vi "runTestScenario.vi"(8 "error in (no error)":errorcluster, 11 "Digital Output Test  in":refnum<class "Digital Output Test.lvclass">) -> (0 "error out":errorcluster, 2 "TestExecution":T1, 3 "Digital Output Test out":refnum<class "Digital Output Test.lvclass">)   [LabVIEW 2015, in "Digital Output Test.lvclass"]
uses:
  Digital Output Test.lvclass
  Typedefs/TestExecution.ctl
  Typedefs/WriteLogMessageInput.ctl
  Typedefs/TestScenarioTypes.ctl
  Typedefs/PassFailTest.ctl
  Digital Output Test.lvclass/Digital Output Test.ctl
  Model/TestLog/ITestLog/ITestLog.lvclass
  Model/ConfigureILCStrategy/IConfigureILCStrategy/IConfigureILCStrategy.lvclass
  Typedefs/ILCBTTypedefs.lvlib
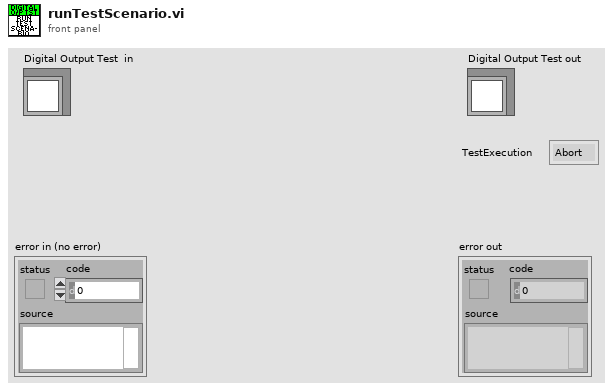
[diagram p1: front panel]
types:
  T1 = typedef "ILCBTTypedefs.lvlib/TestExecution.ctl" = enum16{"Abort", "Continue"}
  T2 = typedef "ILCBTTypedefs.lvlib/WriteLogMessageInput.ctl" = cluster{"Test Scenario":T3, "Description":string, "Actual Value":string, "Data File":string, "Result":T4}
  T3 = typedef "ILCBTTypedefs.lvlib/TestScenarioTypes.ctl" = enum16{"+3.3VA Supply Test", "+3.3VD Supply Test", "+5VA Supply Test", "+5VD Supply Test", "Unique ID Test", "TEDS Status Test", "LIMSW1_TTL Low Test", "LIMSW1_TTL High Test", "LIMSW2_TTL Low Test", "LIMSW2_TTL High Test", "Tachometer Test", "SSR_TTL Low Test", "SSR_TTL High Test", "SM_CW Low Test", "SM_CW High Test", "SM_CCW Low Test", "SM_CCW High Test", "SM_GPI Low Test", "SM_GPI High Test", "CW Motion Without Limit Test", "CW Motion With Limit Test", "CW Motion With Limit Interruption Test", "CW Motion on CCW Limit Test", "CCW Motion Without Limit Test", "CCW Motion With Limit Test", "CCW Motion With Limit Interruption Test", "CCW Motion on CW Limit Test", "RS232-TXD Low Test", "RS232-TXD High Test", "RS232-RTS Low Test", "RS232-RTS High Test", "RS232-RXD Low Test", "RS232-RXD High Test", "RS232-CTS Low Test", "RS232-CTS High Test", "Out_SS Low Test", "Out_SS High Test", "Out_SDI Low Test", "Out_SDI High Test", "Out_SCLK Low Test", "Out_SCLK High Test", "Reset Low Test", "Reset High Test", "1 Channel ADC Test", "3 Channel ADC Test", "5 Channel ADC Test", "Vref Test", "ROT Test", "DAC1 Test", "DAC2 Test", "DAC3 Test", "DAC4 Test", "BIAS Test", "EXC1 Test", "EXC2 Test", "EXC3 Test", "EXC4 Test"}
  T4 = typedef "ILCBTTypedefs.lvlib/PassFailTest.ctl" = enum16{"Fail", "Pass", "NA"}
  T5 = typedef "ILCBTTypedefs.lvlib/Digital Signal Level.ctl" = enum16{"Low", "High"}
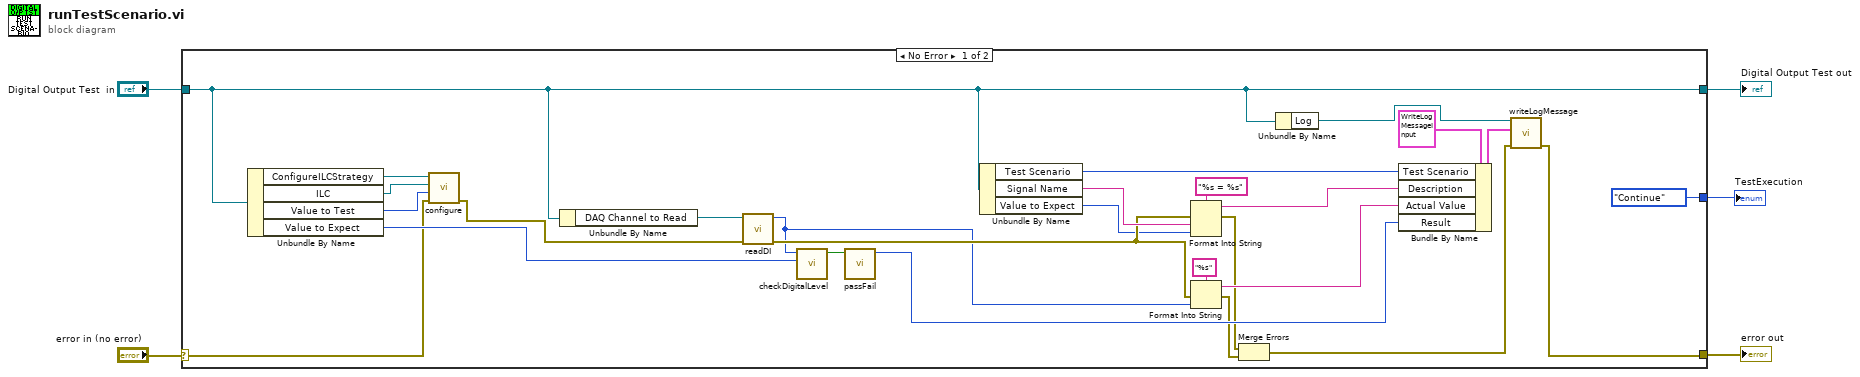
[diagram p0: block diagram]
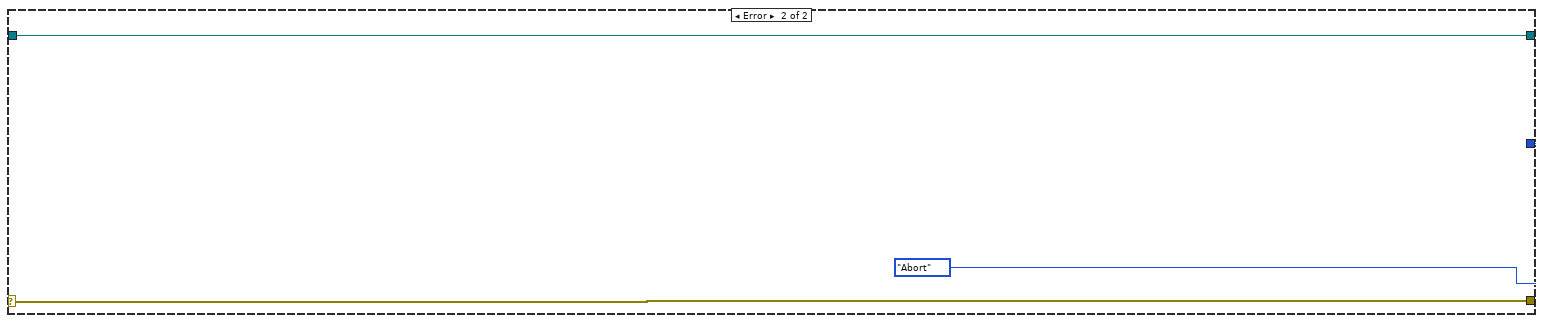
[diagram p2: hidden frame]
diagram:
  n1 = case shown="No Error" "error in (no error)" {
    selector: "error in (no error)" -> [w6 w35]
    tunnel: [w32 w35] -> w4
    tunnel: [TestExecution."Continue" ("TestExecution") TestExecution."Abort" ("TestExecution")] -> w3
    tunnel: "Digital Output Test  in" -> [w8 w33]
    tunnel: [w8 w33] -> w1
    frame No Error {
      n2 = Unbundle By Name(w8) -> ("ConfigureILCStrategy"=w29:refnum<class "IConfigureILCStrategy.lvclass">, "ILC"=w30:refnum<class "ILC.lvclass">, "Value to Test"=w14:u16, "Value to Expect"=w12:T5)
      n3 = call-dynamic "configure.vi"("error in (no error)"=w6, "Value"=w14, "ILC"=w30, "IConfigureILCStrategy in"=w29) -> ("error out"=w13:errorcluster)  [unwired: 6 in, 1 out]
      n4 = Unbundle By Name(w8) -> ("DAQ Channel to Read"=w28:refnum<k21>)
      n5 = call "readDI.vi"("error in (no error)"=w13, "DAQ Channel To Read"=w28) -> ("error out"=w11:errorcluster, "Digital Signal Level"=w9:T5)  [unwired: 8 in]
      n6 = call "checkDigitalLevel.vi"("Expected"=w12, "Actual"=w9) -> ("Pass?"=w27:bool)  [unwired: 9 in]
      n7 = call "passFail.vi"("Boolean"=w27) -> ("Result"=w19:T4)  [unwired: 10 in]
      n8 = Unbundle By Name(w8) -> ("Test Scenario"=w20:T3, "Signal Name"=w25:string, "Value to Expect"=w10:T5)
      n9 = Format Into String(format string="%s = %s", error in=w11, w25, w10) -> (resulting string=w21:string, error out=w17:errorcluster)  [unwired: 1 in]
      n10 = Format Into String(format string="%s", error in=w11, w9) -> (resulting string=w22:string, error out=w18:errorcluster)  [unwired: 1 in]
      n11 = Merge Errors(w17, w18) -> (w16:errorcluster)
      n12 = Unbundle By Name(w8) -> ("Log"=w7:refnum<class "ITestLog.lvclass">)
      n13 = Bundle By Name(cluster=T2 {"Test Scenario"=enum."+3.3VA Supply Test", "Description"="", "Actual Value"="", "Data File"="", "Result"=enum."Fail"} ("WriteLogMessageInput"), "Test Scenario"=w20, "Description"=w21, "Actual Value"=w22, "Result"=w19) -> (w23:T2)
      n14 = call-dynamic "writeLogMessage.vi"("error in (no error)"=w16, "WriteLogMessageInput"=w23, "ITestLog in"=w7) -> ("error out"=w32:errorcluster)  [unwired: 7 in, 1 out]
    }
    frame Error {
    }
  }
  "Digital Output Test out" <- w1
  "error out" <- w4
  "TestExecution" <- w3
